vi "control_esp.vi"() -> ()   [LabVIEW 2018]
uses:
  <vilib>/Utility/file.llb/Write Delimited Spreadsheet (I64).vi
panel:
  in  "Cluster":cluster{"type":string, "content":string}={"type"="get_binary_image", "content"="image"}
  out "error out":errorcluster={"status"=TRUE, "code"=-375003, "source"="Unflatten From JSON in control_esp.vi"}
  out "new picture":picture
  in  "header size":i8=10
  in  "Port 2":u16=1234
  in  "string 8":string="9"
  in  "string 7":string="1"
  in  "string 6":string="168"
  in  "string 5":string="192"
  in  "Backward":bool
  in  "Left":bool
  in  "Forward":bool
  in  "Right":bool
  in  "Port":u16=1234
  in  "string 4":string
  in  "string 3":string
  in  "string 2":string="168"
  in  "string":string="192"
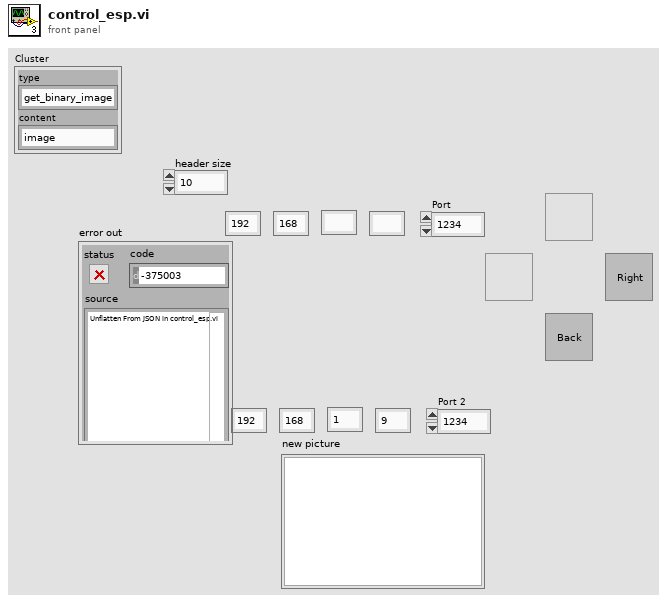
[diagram p1: front panel]
types:
  T1 = typedef "imagedata.ctl" = cluster{"image type":i32, "image depth":i32, "image":u8[], "mask":u8[], "colors":u32[], "Rectangle":cluster{"left":i16, "top":i16, "right":i16, "bottom":i16}}
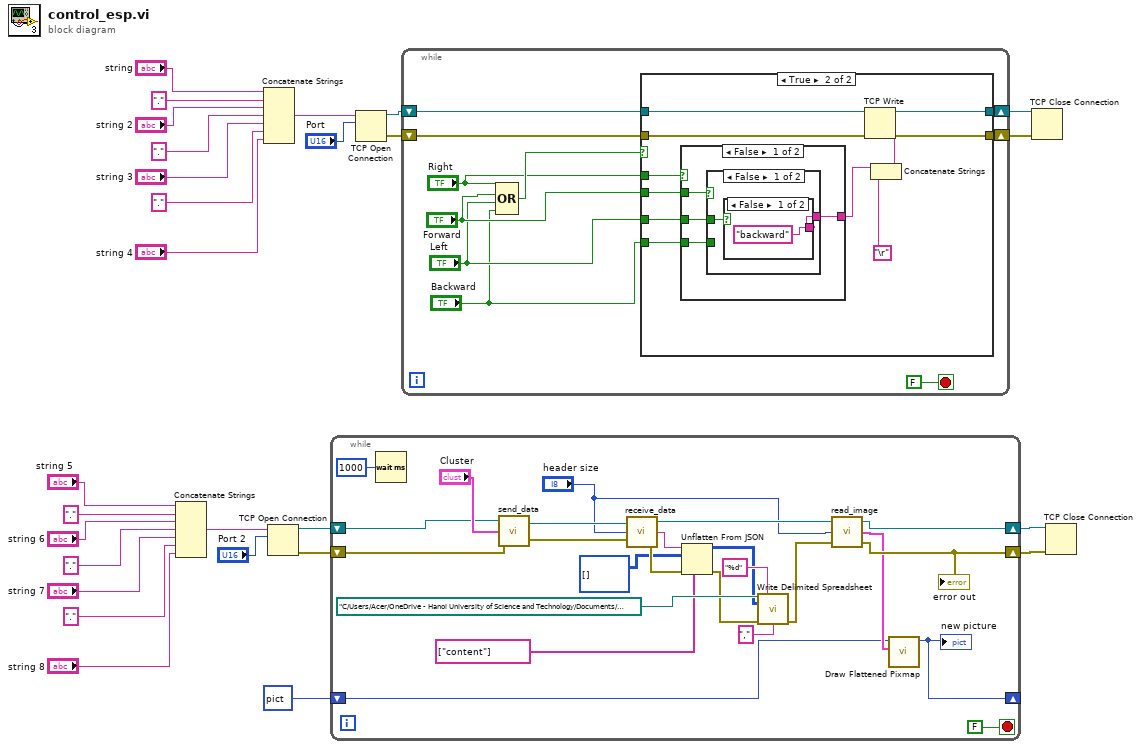
[diagram p0: block diagram]
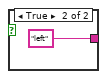
[diagram p3: hidden frame]
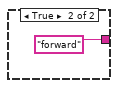
[diagram p4: hidden frame]
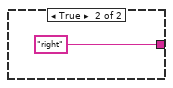
[diagram p5: hidden frame]
diagram:
  n1 = Concatenate Strings("string 5", ".", "string 6", ".", "string 7", ".", "string 8") -> (w20:string)
  n2 = Concatenate Strings("string", ".", "string 2", ".", "string 3", ".", "string 4") -> (w6:string)
  n3 = TCP Open Connection(address=w20, remote port or service name="Port 2") -> (connection ID=w18:refnum<k5>, error out=w17:errorcluster)  [unwired: 3 in]
  n4 = while {
    shift-right: [w34] -> w16
    shift-left: w18 -> [w50]
    shift-right: [w33] -> w15
    shift-left: w17 -> [w49]
    shift-right: [w30] -> _
    shift-left: picture data[5B] ("picture") -> [w31]
    stop <- FALSE stop-if-true
    n5 = Wait (ms)(milliseconds to wait=u32 1000) -> ()  [unwired: 1 out]
    n6 = call "send_data.vi"("error in"=w49, "Cluster"="Cluster", "connection ID"=w50) -> ("error out"=w47:errorcluster, "connection ID out"=w48:refnum<k5>)  [unwired: 1 in]
    n7 = call "receive_data.vi"("error in"=w47, "header size"="header size", "connection ID"=w48) -> ("error out"=w44:errorcluster, "data out"=w45:string, "connection ID out"=w37:refnum<k5>)
    n8 = Unflatten From JSON(path=string[] ["content"], JSON string=w45, type and defaults=i16[][] [], error in (no error)=w44) -> (value=w38:i16[][], error out=w43:errorcluster)  [unwired: 3 in]
    n9 = call-poly <vilib>:"Write Delimited Spreadsheet.vi"("file path (dialog if empty)"=path "C:/Users/Acer/OneDrive - Hanoi University of Science and Technology/Documents/LabViewProject/Project/labview/data.csv", "format (%d)"="%d" ("format (%.3f)"), "2D data"=w38, "error in (no error)"=w43, "delimiter (\\t)"="," ("delimiter (\\t)")) -> ("error out"=w35:errorcluster)  [unwired: 9 in, 1 out]
    n10 = call "read_image.vi"("error in"=w35, "header size"="header size", "connection ID"=w37) -> ("error out"=w33:errorcluster, "image data"=w32:T1, "connection ID out"=w34:refnum<k5>)
    "error out" <- w33
    n11 = call <vilib>:"Draw Flattened Pixmap.vi"("image data"=w32, "picture"=w31) -> ("new picture"=w30:picture)  [unwired: 7 in]
    "new picture" <- w30
  }
  n12 = TCP Open Connection(address=w6, remote port or service name="Port") -> (connection ID=w5:refnum<k5>, error out=w2:errorcluster)  [unwired: 3 in]
  n13 = while {
    shift-right: [w60] -> w4
    shift-left: w5 -> [w61]
    shift-right: [w59] -> w3
    shift-left: w2 -> [w58]
    stop <- FALSE stop-if-true
    n14 = Compound Arithmetic op=OR("Right", "Forward", "Left", "Backward") -> (w57:bool)
    n15 = case shown="True" w57 {
      tunnel: w61 -> [w63 w74]
      tunnel: [w63 w73] -> w60
      tunnel: [w62 w72] -> w59
      tunnel: w58 -> [w62 w71]
      tunnel: "Right" -> [_ w69]
      tunnel: "Forward" -> [_ w67]
      tunnel: "Left" -> [_ w66]
      tunnel: "Backward" -> [_ w65]
      frame False {
      }
      frame True {
        n16 = case shown="False" w69 {
          tunnel: [w77 "right"] -> w68
          tunnel: w67 -> [w78 _]
          tunnel: w66 -> [w76 _]
          tunnel: w65 -> [w75 _]
          frame False {
            n17 = case shown="False" w78 {
              tunnel: [w79 "forward"] -> w77
              tunnel: w76 -> [w80 _]
              tunnel: w75 -> [_ _]
              frame False {
                n18 = case shown="False" w80 {
                  tunnel: ["backward" "left"] -> w79
                  frame False {
                  }
                  frame True {
                  }
                }
              }
              frame True {
              }
            }
          }
          frame True {
          }
        }
        n19 = Concatenate Strings(w68, "\r") -> (w64:string)
        n20 = TCP Write(connection ID=w74, data in=w64, error in (no error)=w71) -> (connection ID out=w73:refnum<k5>, error out=w72:errorcluster)  [unwired: 1 in, 1 out]
      }
    }
  }
  n21 = TCP Close Connection(connection ID=w4, error in (no error)=w3) -> ()  [unwired: 1 in, 2 out]
  n22 = TCP Close Connection(connection ID=w16, error in (no error)=w15) -> ()  [unwired: 1 in, 2 out]
